vi "VIP_Pre-Uninstall Custom Action.vi"(10 "Variant":variant) -> (0 "error out":errorcluster)   [LabVIEW 2020]
uses:
  <vilib>/Utility/sysdir.llb/System Directory Type.ctl
  <userlib>/_OpenG.lib/file/file.llb/openg_file.lvlib
  <userlib>/_OpenG.lib/file/file.llb/Build Path - Traditional__ogtk.vi
  <userlib>/_OpenG.lib/lvzip/lvzip.llb/subVI/ZLIB Extract All Files To Dir (Path)__ogtk.vi
panel:
  # "pre uninstall"
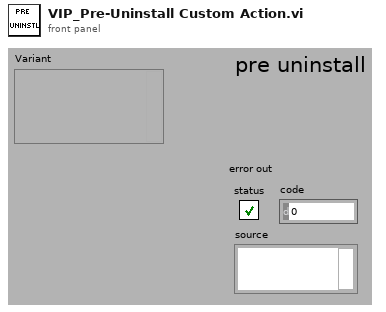
[diagram p1: front panel]
types:
  T1 = typedef "System Directory Type.ctl" = i32
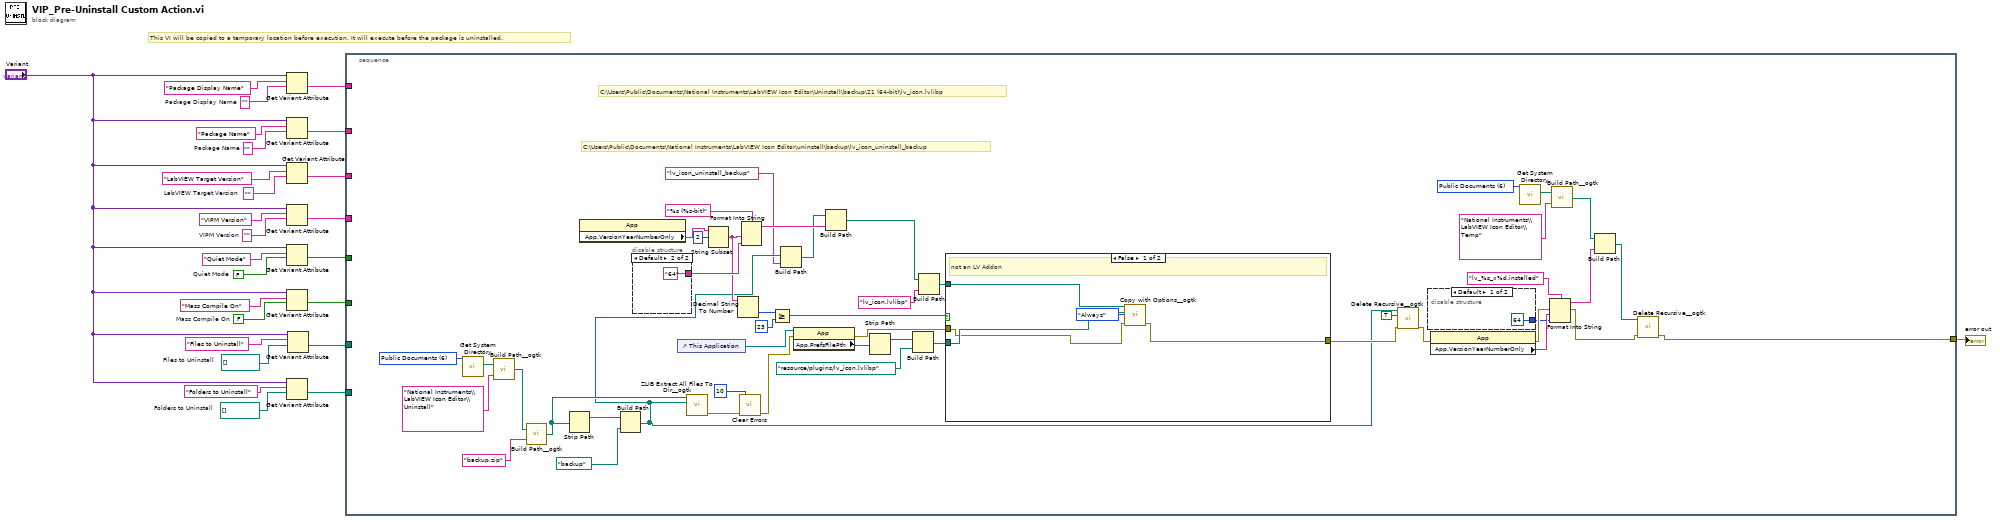
[diagram p0: block diagram]
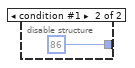
[diagram p2: hidden frame]
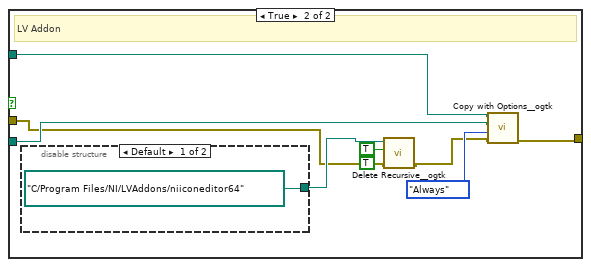
[diagram p3: hidden frame]
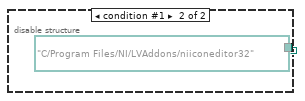
[diagram p4: hidden frame]
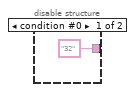
[diagram p5: hidden frame]
diagram:
  w11 = path[] []  # Folders to Uninstall
  w14 = path[] []  # Files to Uninstall
  w15 = FALSE  # Mass Compile On
  w16 = ""  # Package Display Name
  w17 = FALSE  # Quiet Mode
  w20 = ""  # VIPM Version
  w22 = ""  # LabVIEW Target Version
  w24 = ""  # Package Name
  # "This VI will be copied to a temporary location before execution. It will execute before the package is uninstalled."
  n1 = Get Variant Attribute(Variant="Variant", name="Package Display Name", default value (empty Variant)=w16) -> (value=w9:string)  [unwired: 1 in, 3 out]
  n2 = Get Variant Attribute(Variant="Variant", name="Package Name", default value (empty Variant)=w24) -> (value=w8:string)  [unwired: 1 in, 3 out]
  n3 = Get Variant Attribute(Variant="Variant", name="LabVIEW Target Version", default value (empty Variant)=w22) -> (value=w7:string)  [unwired: 1 in, 3 out]
  n4 = Get Variant Attribute(Variant="Variant", name="VIPM Version", default value (empty Variant)=w20) -> (value=w6:string)  [unwired: 1 in, 3 out]
  n5 = Get Variant Attribute(Variant="Variant", name="Quiet Mode", default value (empty Variant)=w17) -> (value=w5:bool)  [unwired: 1 in, 3 out]
  n6 = Get Variant Attribute(Variant="Variant", name="Mass Compile On", default value (empty Variant)=w15) -> (value=w4:bool)  [unwired: 1 in, 3 out]
  n7 = Get Variant Attribute(Variant="Variant", name="Folders to Uninstall", default value (empty Variant)=w11) -> (value=w2:path[])  [unwired: 1 in, 3 out]
  n8 = Get Variant Attribute(Variant="Variant", name="Files to Uninstall", default value (empty Variant)=w14) -> (value=w3:path[])  [unwired: 1 in, 3 out]
  n9 = stacked-sequence {
    tunnel: w9 -> [_]
    tunnel: w8 -> [_]
    tunnel: w7 -> [_]
    tunnel: w6 -> [_]
    tunnel: w5 -> [_]
    tunnel: w4 -> [_]
    tunnel: w3 -> [_]
    tunnel: w2 -> [_]
    tunnel: [w27] -> w1
    frame #0 {
      w40 = T1 6 items=["User Home"=0, "User Desktop"=1, "User Documents"=2, "User Application Data"=3, "User Preferences"=4, "User Temporary"=5, "Public Documents"=6, "Public Application Data"=7, "Public Preferences"=8, "Public Cache"=13, "System Core Libraries"=9, "System Installed Libraries"=10, "Application Files"=11, "Boot Volume Root"=12] ("system directory type")
      w55 = T1 6 items=["User Home"=0, "User Desktop"=1, "User Documents"=2, "User Application Data"=3, "User Preferences"=4, "User Temporary"=5, "Public Documents"=6, "Public Application Data"=7, "Public Preferences"=8, "Public Cache"=13, "System Core Libraries"=9, "System Installed Libraries"=10, "Application Files"=11, "Boot Volume Root"=12] ("system directory type")
      # "C:\\Users\\Public\\Documents\\National Instruments\\LabVIEW Icon Editor\\uninstall\\backup\\lv_icon_uninstall_backup"
      # "C:\\Users\\Public\\Documents\\National Instruments\\LabVIEW Icon Editor\\Uninstall\\backup\\21 (64-bit)\\lv_icon.lvlibp"
      n10 = call <vilib>:"Get System Directory.vi"("system directory type"=w55) -> ("system directory"=w54:path)  [unwired: 10 in]
      n11 = call-poly <userlib>:"Build Path__ogtk.vi"("name or relative path"="National Instruments\\LabVIEW Icon Editor\\Uninstall", "base path"=w54) -> ("appended path"=w51:path)
      n12 = call-poly <userlib>:"Build Path__ogtk.vi"("name or relative path"="backup.zip", "base path"=w51) -> ("appended path"=w46:path)
      n13 = Strip Path(path=w46) -> (stripped path=w50:path)  [unwired: 1 out]
      n14 = property class="App"() -> ("App.VersionYearNumberOnly"=w59:string)  [unwired: 2 in, 2 out]
      n15 = Build Path(base path=w50, name or relative path=path "backup") -> (appended path=w32:path)
      n16 = disable-structure shown="Default" {
        disable-tunnel: ["32" "64"] -> w72
        frame condition #0 {
        }
        frame condition #1 (active) {
        }
      }
      n17 = control-ref of="This Application"() -> (w56:refnum<vi>)
      n18 = call-poly <userlib>:"ZLIB Extract All Files To Dir__ogtk.vi"("destination directory (archive name without ending)"=w32, "archive name (file dialog)"=w46) -> ("error out"=w35:errorcluster)  [unwired: 7 in, 2 out]
      n19 = String Subset(string=w59, offset (0)=2) -> (substring=w58:string)  [unwired: 1 in]
      n20 = Decimal String To Number(string=w58) -> (number=w70:i32)  [unwired: 2 in, 1 out]
      n21 = call <vilib>:"Clear Errors.vi"("error in (no error)"=w35, "specific error code to clear (0: all)"=10) -> ("error out"=w34:errorcluster)  [unwired: 4 in, 1 out]
      n22 = Format Into String(format string="%s (%s-bit)", w58, w72) -> (resulting string=w62:string)  [unwired: 2 in, 1 out]
      n23 = Greater Or Equal?(x=w70, y=23) -> (x >= y?=w64:bool)
      n24 = Build Path(base path=w32, name or relative path="lv_icon_uninstall_backup" ("resulting string")) -> (appended path=w31:path)
      n25 = property class="App"(reference=w56, error in=w34) -> (error out=w61:errorcluster, "App.PrefsFilePth"=w71:path)  [unwired: 1 out]
      n26 = Build Path(base path=w31, name or relative path=w62) -> (appended path=w57:path)
      n27 = Strip Path(path=w71) -> (stripped path=w68:path)  [unwired: 1 out]
      n28 = Build Path(base path=w68, name or relative path=path "resource/plugins/lv_icon.lvlibp") -> (appended path=w66:path)
      n29 = Build Path(base path=w57, name or relative path="lv_icon.lvlibp" ("resulting string")) -> (appended path=w63:path)
      n30 = case shown="False" w64 {
        tunnel: [w76 w89] -> w45
        tunnel: w66 -> [w78 w86]
        tunnel: w63 -> [w79 w87]
        tunnel: w61 -> [w77 w84]
        frame False {
          # "not an LV Addon"
          n31 = call <userlib>:"Copy with Options__ogtk.vi"("error in (no error)"=w77, "Replace Mode (Never)"=enum16{"Never", "Always", "If Newer"}."Always", "target path"=w78, "source path"=w79) -> ("error out"=w76:errorcluster)  [unwired: 6 in, 1 out]
        }
        frame True {
          # "LV Addon"
          n32 = disable-structure shown="Default" {
            disable-tunnel: [path "C:/Program Files/NI/LVAddons/niiconeditor64" ("Destination[i] Paths (Absolute)") path "C:/Program Files/NI/LVAddons/niiconeditor32" ("Destination[i] Paths (Absolute)")] -> w85
            frame condition #0 (active) {
            }
            frame condition #1 {
            }
          }
          n33 = call <userlib>:"Delete Recursive__ogtk.vi"("error in (no error)"=w84, "Ignore Read-Only? (FALSE)"=TRUE, "Recursive? (FALSE)"=TRUE, "Path"=w85) -> ("error out"=w83:errorcluster)  [unwired: 6 in, 1 out]
          n34 = call <userlib>:"Copy with Options__ogtk.vi"("error in (no error)"=w83, "Replace Mode (Never)"=enum16{"Never", "Always", "If Newer"}."Always", "target path"=w86, "source path"=w87) -> ("error out"=w89:errorcluster)  [unwired: 6 in, 1 out]
        }
      }
      n35 = call <userlib>:"Delete Recursive__ogtk.vi"("error in (no error)"=w45, "Recursive? (FALSE)"=TRUE, "Path"=w32) -> ("error out"=w44:errorcluster)  [unwired: 7 in, 1 out]
      n36 = disable-structure shown="Default" {
        disable-tunnel: [64 ("code") 86 ("code")] -> w38
        frame condition #0 (active) {
        }
        frame condition #1 {
        }
      }
      n37 = property class="App"(error in=w44) -> (error out=w47:errorcluster, "App.VersionYearNumberOnly"=w39:string)  [unwired: 1 in, 1 out]
      n38 = call <vilib>:"Get System Directory.vi"("system directory type"=w40) -> ("system directory"=w41:path)  [unwired: 10 in]
      n39 = Format Into String(format string="lv_%s_x%d.installed", error in=w47, w39, w38) -> (resulting string=w37:string, error out=w28:errorcluster)  [unwired: 1 in]
      n40 = call-poly <userlib>:"Build Path__ogtk.vi"("name or relative path"="National Instruments\\LabVIEW Icon Editor\\Temp", "base path"=w41) -> ("appended path"=w36:path)
      n41 = Build Path(base path=w36, name or relative path=w37) -> (appended path=w29:path)
      n42 = call <userlib>:"Delete Recursive__ogtk.vi"("error in (no error)"=w28, "Path"=w29) -> ("error out"=w27:errorcluster)  [unwired: 8 in, 1 out]
    }
  }
  "error out" <- w1
